vi "Assemble Rectifier Setting Changes for PLC.vi"(6 "Num Steps":i32, 7 "Rect Number":i32=1, 8 "error In":errorcluster, 9 "Reverse Current Multiplier":dbl=3.0, 10 "message queue in":T1, 11 "MulticolumnListbox in":refnum<vi>) -> (0 "Right Anode Mins":dbl, 1 "Left Anode Mins":dbl, 2 "Right AmpMin":dbl, 3 "Left AmpMin":dbl, 4 "error out":errorcluster)   [LabVIEW 2019]
uses:
  <vilib>/NI/AMC/Message Queue.ctl
  <vilib>/NI/AMC/Message.ctl
  <vilib>/NI/Tools/Keyed Array/KeyedArray.ctl
  <vilib>/NI/Current Value Table/Type Defs/Single Tag.ctl
  <vilib>/NI/Current Value Table/Type Defs/Data Types.ctl
  <vilib>/NI/AMC/Create Single Message.vi
  <vilib>/NI/AMC/Update Message Routing Info.vi
  <vilib>/NI/AMC/Send Message.vi
  <vilib>/NI/AMC/AMC.lvlib
  <vilib>/NI/Current Value Table/Current Value Table.lvlib
  <vilib>/NI/Tools/Keyed Array/Tools_KeyedArray.lvlib
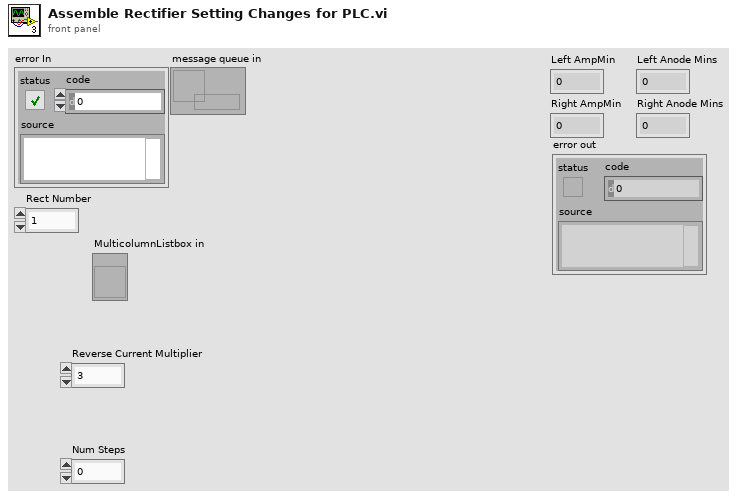
[diagram p1: front panel]
types:
  T1 = typedef "AMC.lvlib/Message Queue.ctl" = refnum<queue>
  T2 = typedef "Current Value Table.lvlib/Data Types.ctl" = enum16{"Double", "Single", "I64", "I32", "I16", "I8", "U64", "U32", "U16", "U8", "String", "Boolean", "Array of U8", "Array of U16", "Array of U32", "Array of U64", "Array of I64", "Array of I32", "Array of I16", "Array of I8", "Array of Double", "Array of Single", "Array of Boolean", "Array of String"}
  T3 = typedef "Current Value Table.lvlib/Single Tag.ctl" = cluster{"Data Type":T2, "Name":string, "Value":string, "Description":string}
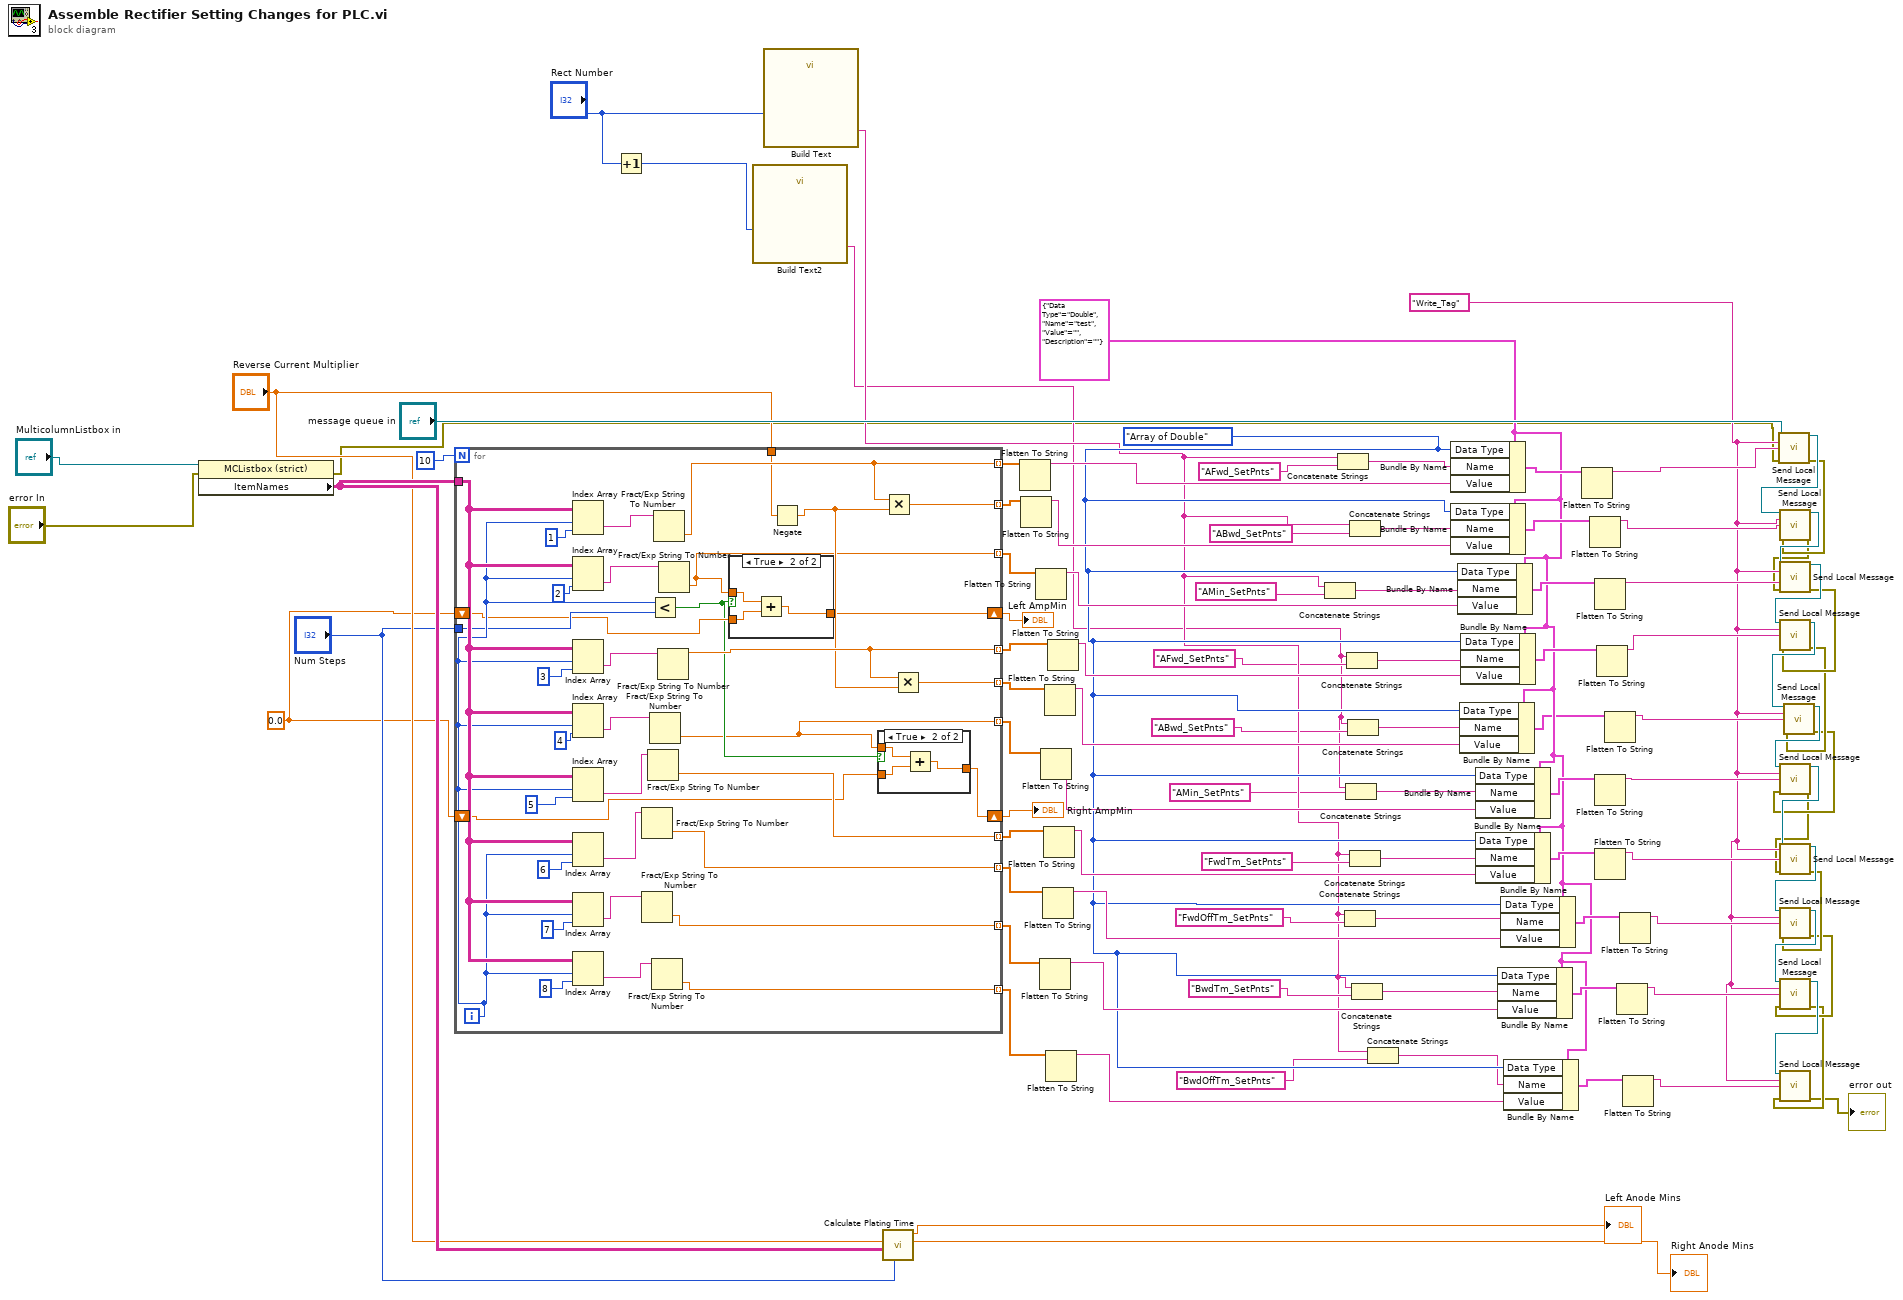
[diagram p0: block diagram]
diagram:
  w15 = 0.0
  w49 = Data_Types."Array of Double" ("Data Type")
  w52 = T3 {"Data Type"=enum."Double", "Name"="test", "Value"="", "Description"=""} ("Tag")
  w44 = "Write_Tag" ("message name")
  n1 = property class="MCListbox (strict)"(reference="MulticolumnListbox in", error in="error In") -> (error out=w13:errorcluster, "ItemNames"=w19:string[][])  [unwired: 1 out]
  n2 = for {
    N: 10 -> [_]
    tunnel: w19 -> [w126]
    tunnel: [w114] -> w96 mode=indexing
    tunnel: [w106] -> w91 mode=indexing
    tunnel: [w112] -> w87 mode=indexing
    tunnel: [w102] -> w82 mode=indexing
    tunnel: [w118] -> w70 mode=indexing
    tunnel: [w117] -> w63 mode=indexing
    tunnel: [w116] -> w57 mode=indexing
    tunnel: [w115] -> w50 mode=indexing
    tunnel: [w113] -> w78 mode=indexing
    tunnel: [w110] -> w76 mode=indexing
    tunnel: "Reverse Current Multiplier" -> [w109]
    tunnel: "Num Steps" -> [w107]
    shift-right: [w104] -> w2
    shift-left: w15 -> [w105]
    shift-right: [w100] -> w1
    shift-left: w15 -> [w101]
    i -> [w108]
    n3 = Index Array(array=w126, index (row)=w108, index (col)=1 ("disabled index (col)")) -> (element=w134:string)
    n4 = Index Array(array=w126, index (row)=w108, index (col)=2 ("disabled index (col)")) -> (element=w125:string)
    n5 = Index Array(array=w126, index (row)=w108, index (col)=3 ("disabled index (col)")) -> (element=w124:string)
    n6 = Index Array(array=w126, index (row)=w108, index (col)=4 ("disabled index (col)")) -> (element=w123:string)
    n7 = Index Array(array=w126, index (row)=w108, index (col)=5 ("disabled index (col)")) -> (element=w122:string)
    n8 = Index Array(array=w126, index (row)=w108, index (col)=6 ("disabled index (col)")) -> (element=w121:string)
    n9 = Index Array(array=w126, index (row)=w108, index (col)=7 ("disabled index (col)")) -> (element=w120:string)
    n10 = Index Array(array=w126, index (row)=w108, index (col)=8 ("disabled index (col)")) -> (element=w119:string)
    n11 = Fract/Exp String To Number(string=w121) -> (number=w117:dbl)  [unwired: 3 in, 1 out]
    n12 = Fract/Exp String To Number(string=w120) -> (number=w116:dbl)  [unwired: 3 in, 1 out]
    n13 = Fract/Exp String To Number(string=w122) -> (number=w118:dbl)  [unwired: 3 in, 1 out]
    n14 = Less?(x=w108, y=w107) -> (x < y?=w103:bool)
    n15 = Fract/Exp String To Number(string=w123) -> (number=w102:dbl)  [unwired: 3 in, 1 out]
    n16 = Fract/Exp String To Number(string=w119) -> (number=w115:dbl)  [unwired: 3 in, 1 out]
    n17 = Fract/Exp String To Number(string=w134) -> (number=w114:dbl)  [unwired: 3 in, 1 out]
    n18 = Fract/Exp String To Number(string=w124) -> (number=w112:dbl)  [unwired: 3 in, 1 out]
    n19 = Fract/Exp String To Number(string=w125) -> (number=w106:dbl)  [unwired: 3 in, 1 out]
    n20 = case shown="True" w103 {
      tunnel: w106 -> [_ w143]
      tunnel: w105 -> [w140 w142]
      tunnel: [w140 w141] -> w104
      frame False {
      }
      frame True {
        n21 = Add(x=w143, y=w142) -> (x+y=w141:dbl)
      }
    }
    n22 = Negate(x=w109) -> (-x=w111:dbl)
    n23 = case shown="True" w103 {
      tunnel: w102 -> [_ w139]
      tunnel: w101 -> [w136 w138]
      tunnel: [w136 w137] -> w100
      frame False {
      }
      frame True {
        n24 = Add(x=w139, y=w138) -> (x+y=w137:dbl)
      }
    }
    n25 = Multiply(x=w114, y=w111) -> (x*y=w113:dbl)
    n26 = Multiply(x=w112, y=w111) -> (x*y=w110:dbl)
  }
  "Left AmpMin" <- w2
  "Right AmpMin" <- w1
  n27 = Increment(x="Rect Number") -> (x+1=w42:i32)
  n28 = call "Build Text2"("Rect1"=w42) -> ("Result"=w21:string)  [unwired: 13 in, 1 out]
  n29 = call "Build Text"("Rect1"="Rect Number") -> ("Result"=w28:string)  [unwired: 13 in, 1 out]
  n30 = call "Calculate Plating Time.vi"("Num Steps"="Num Steps", "ItemNames"=w19, "Reverse Current Multiplier"="Reverse Current Multiplier") -> ("Right Anode Time"=→"Right Anode Mins":dbl, "Left Anode Time"=→"Left Anode Mins":dbl)  [unwired: 7 in]
  n31 = Flatten To String(anything=w96) -> (data string=w94:string)  [unwired: 3 in, 2 out]
  n32 = Flatten To String(anything=w78) -> (data string=w77:string)  [unwired: 3 in, 2 out]
  n33 = Flatten To String(anything=w91) -> (data string=w90:string)  [unwired: 3 in, 2 out]
  n34 = Flatten To String(anything=w57) -> (data string=w58:string)  [unwired: 3 in, 2 out]
  n35 = Flatten To String(anything=w82) -> (data string=w81:string)  [unwired: 3 in, 2 out]
  n36 = Flatten To String(anything=w63) -> (data string=w62:string)  [unwired: 3 in, 2 out]
  n37 = Flatten To String(anything=w70) -> (data string=w69:string)  [unwired: 3 in, 2 out]
  n38 = Flatten To String(anything=w76) -> (data string=w71:string)  [unwired: 3 in, 2 out]
  n39 = Flatten To String(anything=w50) -> (data string=w51:string)  [unwired: 3 in, 2 out]
  n40 = Flatten To String(anything=w87) -> (data string=w86:string)  [unwired: 3 in, 2 out]
  n41 = Concatenate Strings(w28, "AMin_SetPnts" ("Name")) -> (w37:string)
  n42 = Concatenate Strings(w28, "AFwd_SetPnts" ("Name")) -> (w41:string)
  n43 = Concatenate Strings(w28, "FwdOffTm_SetPnts" ("Name")) -> (w33:string)
  n44 = Concatenate Strings(w21, "AMin_SetPnts" ("Name")) -> (w22:string)
  n45 = Concatenate Strings(w21, "AFwd_SetPnts" ("Name")) -> (w25:string)
  n46 = Concatenate Strings(w21, "ABwd_SetPnts" ("Name")) -> (w24:string)
  n47 = Concatenate Strings(w28, "ABwd_SetPnts" ("Name")) -> (w39:string)
  n48 = Concatenate Strings(w28, "FwdTm_SetPnts" ("Name")) -> (w35:string)
  n49 = Concatenate Strings(w28, "BwdTm_SetPnts" ("Name")) -> (w31:string)
  n50 = Concatenate Strings(w28, "BwdOffTm_SetPnts" ("Name")) -> (w27:string)
  n51 = Bundle By Name(cluster=w52, "Data Type"=w49, "Name"=w41, "Value"=w94) -> (w93:T3)
  n52 = Bundle By Name(cluster=w52, "Data Type"=w49, "Name"=w39, "Value"=w77) -> (w75:T3)
  n53 = Bundle By Name(cluster=w52, "Data Type"=w49, "Name"=w37, "Value"=w90) -> (w89:T3)
  n54 = Bundle By Name(cluster=w52, "Data Type"=w49, "Name"=w24, "Value"=w71) -> (w48:T3)
  n55 = Bundle By Name(cluster=w52, "Data Type"=w49, "Name"=w25, "Value"=w86) -> (w85:T3)
  n56 = Bundle By Name(cluster=w52, "Data Type"=w49, "Name"=w22, "Value"=w81) -> (w80:T3)
  n57 = Bundle By Name(cluster=w52, "Data Type"=w49, "Name"=w35, "Value"=w69) -> (w68:T3)
  n58 = Bundle By Name(cluster=w52, "Data Type"=w49, "Name"=w31, "Value"=w58) -> (w60:T3)
  n59 = Bundle By Name(cluster=w52, "Data Type"=w49, "Name"=w33, "Value"=w62) -> (w65:T3)
  n60 = Bundle By Name(cluster=w52, "Data Type"=w49, "Name"=w27, "Value"=w51) -> (w55:T3)
  n61 = Flatten To String(anything=w93) -> (data string=w92:string)  [unwired: 3 in, 2 out]
  n62 = Flatten To String(anything=w75) -> (data string=w72:string)  [unwired: 3 in, 2 out]
  n63 = Flatten To String(anything=w89) -> (data string=w88:string)  [unwired: 3 in, 2 out]
  n64 = Flatten To String(anything=w80) -> (data string=w79:string)  [unwired: 3 in, 2 out]
  n65 = Flatten To String(anything=w68) -> (data string=w66:string)  [unwired: 3 in, 2 out]
  n66 = Flatten To String(anything=w85) -> (data string=w83:string)  [unwired: 3 in, 2 out]
  n67 = Flatten To String(anything=w48) -> (data string=w45:string)  [unwired: 3 in, 2 out]
  n68 = Flatten To String(anything=w60) -> (data string=w59:string)  [unwired: 3 in, 2 out]
  n69 = Flatten To String(anything=w65) -> (data string=w64:string)  [unwired: 3 in, 2 out]
  n70 = Flatten To String(anything=w55) -> (data string=w54:string)  [unwired: 3 in, 2 out]
  n71 = call <vilib>:"Send Local Message.vi"("message queue in"="message queue in", "message name"=w44, "message value"=w92, "error in"=w13) -> ("message queue out"=w74:T1, "error out"=w12:errorcluster)  [unwired: 9 in, 1 out]
  n72 = call <vilib>:"Send Local Message.vi"("message queue in"=w74, "message name"=w44, "message value"=w72, "error in"=w12) -> ("message queue out"=w73:T1, "error out"=w11:errorcluster)  [unwired: 9 in, 1 out]
  n73 = call <vilib>:"Send Local Message.vi"("message queue in"=w73, "message name"=w44, "message value"=w88, "error in"=w11) -> ("message queue out"=w84:T1, "error out"=w10:errorcluster)  [unwired: 9 in, 1 out]
  n74 = call <vilib>:"Send Local Message.vi"("message queue in"=w84, "message name"=w44, "message value"=w83, "error in"=w10) -> ("message queue out"=w47:T1, "error out"=w9:errorcluster)  [unwired: 9 in, 1 out]
  n75 = call <vilib>:"Send Local Message.vi"("message queue in"=w47, "message name"=w44, "message value"=w45, "error in"=w9) -> ("message queue out"=w46:T1, "error out"=w8:errorcluster)  [unwired: 9 in, 1 out]
  n76 = call <vilib>:"Send Local Message.vi"("message queue in"=w46, "message name"=w44, "message value"=w79, "error in"=w8) -> ("message queue out"=w67:T1, "error out"=w7:errorcluster)  [unwired: 9 in, 1 out]
  n77 = call <vilib>:"Send Local Message.vi"("message queue in"=w67, "message name"=w44, "message value"=w66, "error in"=w7) -> ("message queue out"=w61:T1, "error out"=w6:errorcluster)  [unwired: 9 in, 1 out]
  n78 = call <vilib>:"Send Local Message.vi"("message queue in"=w61, "message name"=w44, "message value"=w64, "error in"=w6) -> ("message queue out"=w56:T1, "error out"=w5:errorcluster)  [unwired: 9 in, 1 out]
  n79 = call <vilib>:"Send Local Message.vi"("message queue in"=w56, "message name"=w44, "message value"=w59, "error in"=w5) -> ("message queue out"=w53:T1, "error out"=w4:errorcluster)  [unwired: 9 in, 1 out]
  n80 = call <vilib>:"Send Local Message.vi"("message queue in"=w53, "message name"=w44, "message value"=w54, "error in"=w4) -> ("error out"=→"error out":errorcluster)  [unwired: 9 in, 2 out]
